vi "_AdjustAndDisplay.vi"(7 "Refs":T2, 9 "Action in":T1 caption="Action", 10 "Display State In in":T3 caption="State", 11 "Data In in":T6) -> (1 "Action out":T1 caption="Action", 2 "Display State In out":T3 caption="State", 3 "Data In out":T6)   [LabVIEW 2017, in "UI_TimeSelector.xctl"]
uses:
  UI_TimeSelector.xctl
  Data.ctl
  State.ctl
  Typedefs/INTERNAL-DATA.ctl
  Interface/DEF-Mode.ctl
  Typedefs/INTERNAL-REFs.ctl
  <vilib>/_xctls/Action.ctl
  <vilib>/_xctls/XControlSupport.lvlib
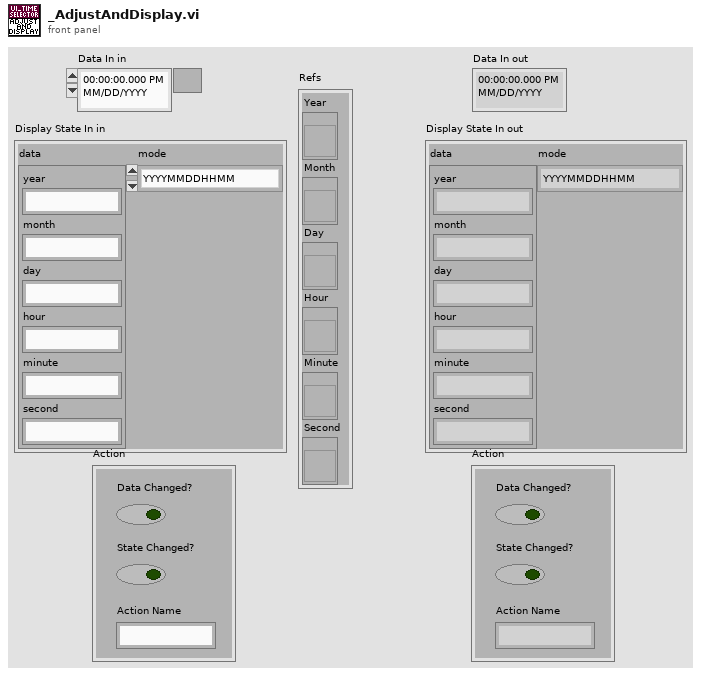
[diagram p1: front panel]
types:
  T1 = typedef "XControlSupport.lvlib/Action.ctl" = cluster{"Data Changed?":bool, "State Changed?":bool, "Action Name":string}
  T2 = typedef "UI_TimeSelector.xctl/INTERNAL-REFs.ctl" = cluster{"Year":refnum<vi>, "Month":refnum<vi>, "Day":refnum<vi>, "Hour":refnum<vi>, "Minute":refnum<vi>, "Second":refnum<vi>}
  T3 = typedef "UI_TimeSelector.xctl/State.ctl" = cluster{"data":T4, "mode":T5}
  T4 = typedef "UI_TimeSelector.xctl/INTERNAL-DATA.ctl" = cluster{"year":string, "month":string, "day":string, "hour":string, "minute":string, "second":string}
  T5 = typedef "UI_TimeSelector.xctl/DEF-Mode.ctl" = enum16{"YYYYMMDDHHMM", "YYYYMMDDHHMMSS", "YYYY", "YYYYMM", "YYYYMMDD", "HHMM", "HHMMSS"}
  T6 = typedef "UI_TimeSelector.xctl/Data.ctl" = timestamp
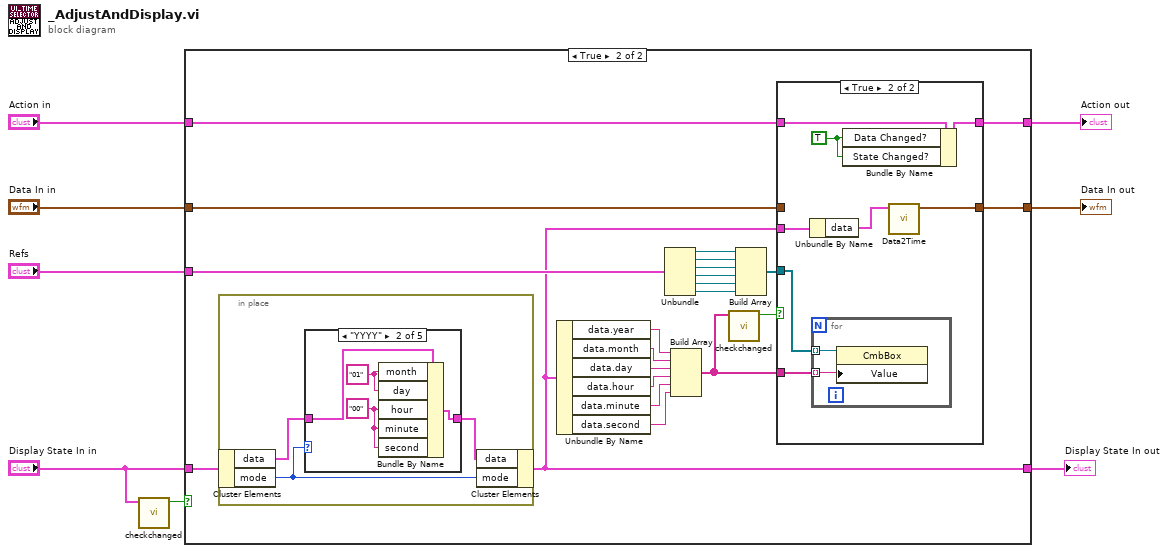
[diagram p0: block diagram]
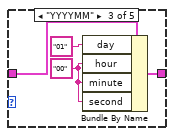
[diagram p5: hidden frame]
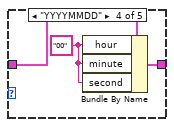
[diagram p6: hidden frame]
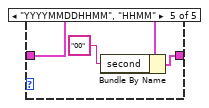
[diagram p7: hidden frame]
diagram:
  n1 = call "checkchanged.vi"("mode"="Display State In in") -> ("Boolean"=w5:bool)  [unwired: 10 in]
  n2 = case shown="True" w5 {
    tunnel: [w11 w14] -> w8
    tunnel: "Refs" -> [_ w33]
    tunnel: "Display State In in" -> [w11 w17]
    tunnel: [w10 w13] -> w4
    tunnel: "Action in" -> [w10 w15]
    tunnel: [w9 w16] -> w2
    tunnel: "Data In in" -> [w9 w12]
    frame False {
    }
    frame True {
      n3 = in-place {
        n4 = in-place-cluster #1(w17) -> ("data"=w47:T4, "mode"=w48:T5)
        n5 = case shown="\"YYYY\"" w48 {
          tunnel: w47 -> [w49 w53 w55 w59 w63]
          tunnel: [w49 w52 w54 w58 w62] -> w46
          frame "YYYYMMDDHHMMSS", "HHMMSS", Default {
          }
          frame "YYYY" {
            w50 = "01" ("hour")
            w51 = "00" ("hour")
            n6 = Bundle By Name(cluster=w53, "month"=w50, "day"=w50, "hour"=w51, "minute"=w51, "second"=w51) -> (w52:T4)
          }
          frame "YYYYMM" {
            w57 = "00" ("hour")
            n7 = Bundle By Name(cluster=w55, "day"="01" ("hour"), "hour"=w57, "minute"=w57, "second"=w57) -> (w54:T4)
          }
          frame "YYYYMMDD" {
            w60 = "00" ("hour")
            n8 = Bundle By Name(cluster=w59, "hour"=w60, "minute"=w60, "second"=w60) -> (w58:T4)
          }
          frame "YYYYMMDDHHMM", "HHMM" {
            n9 = Bundle By Name(cluster=w63, "second"="00" ("hour")) -> (w62:T4)
          }
        }
        n10 = in-place-cluster #1("data"=w46, "mode"=w48) -> (w14:T3)
      }
      n11 = Unbundle By Name(w14) -> ("data.year"=w26:string, "data.month"=w25:string, "data.day"=w24:string, "data.hour"=w23:string, "data.minute"=w22:string, "data.second"=w21:string)
      n12 = Unbundle(w33) -> ("Year"=w32:refnum<vi>, "Month"=w31:refnum<vi>, "Day"=w30:refnum<vi>, "Hour"=w29:refnum<vi>, "Minute"=w28:refnum<vi>, "Second"=w27:refnum<vi>)
      n13 = Build Array(w26, w25, w24, w23, w22, w21) -> (w19:string[])
      n14 = call "checkchanged.vi"("mode"=w19) -> ("Boolean"=w18:bool)  [unwired: 10 in]
      n15 = Build Array(w32, w31, w30, w29, w28, w27) -> (w20:refnum<vi>[])
      n16 = case shown="True" w18 {
        tunnel: w20 -> [_ w43]
        tunnel: w19 -> [_ w42]
        tunnel: [w35 w41] -> w16
        tunnel: w15 -> [w34 w38]
        tunnel: w14 -> [_ w40]
        tunnel: [w34 w37] -> w13
        tunnel: w12 -> [w35 _]
        frame False {
        }
        frame True {
          w36 = TRUE ("Data Changed?")
          n17 = Unbundle By Name(w40) -> ("data"=w39:T4)
          n18 = for {
            tunnel: w43 -> [w45] mode=indexing
            tunnel: w42 -> [w44] mode=indexing
            n19 = property class="CmbBox"(reference=w45, "Value"=w44) -> ()  [unwired: 1 in, 2 out]
          }
          n20 = Bundle By Name(cluster=w38, "Data Changed?"=w36, "State Changed?"=w36) -> (w37:T1)
          n21 = call "Data2Time.vi"("data"=w39) -> ("Time"=w41:timestamp)  [unwired: 10 in]
        }
      }
    }
  }
  "Data In out" <- w2
  "Display State In out" <- w8
  "Action out" <- w4
